vi "WaitOnStopMove.vi"(8 "error in (no error)":errorcluster, 9 "ignore previous (F)":bool, 10 "timeout in ms (-1)":i32, 11 "Game in":refnum<class "Game.lvclass">) -> (0 "error out":errorcluster, 2 "timed out?":bool, 3 "Game out":refnum<class "Game.lvclass">)   [LabVIEW 2019, in "RT_Game.lvlib" / "Game.lvclass"]
uses:
  Game.lvclass
  Game.lvclass/Game.ctl
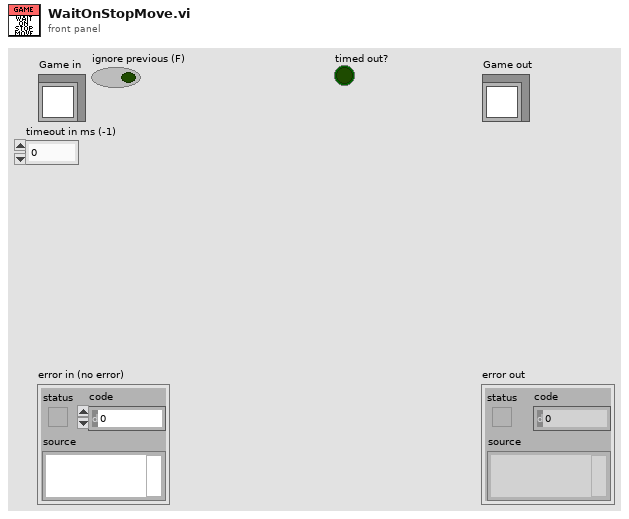
[diagram p1: front panel]
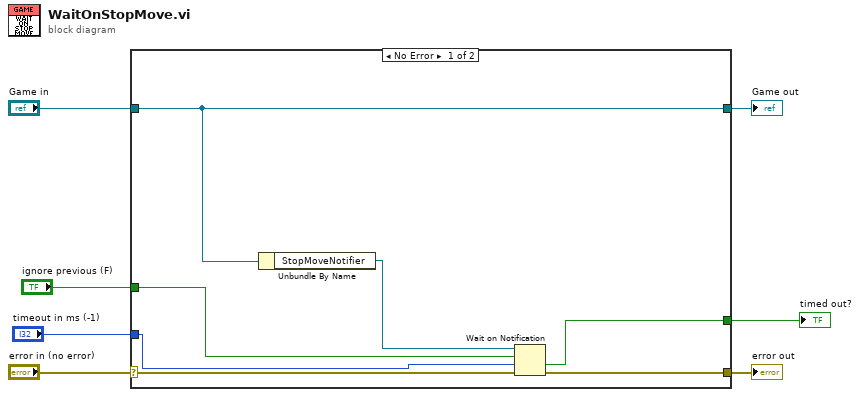
[diagram p0: block diagram]
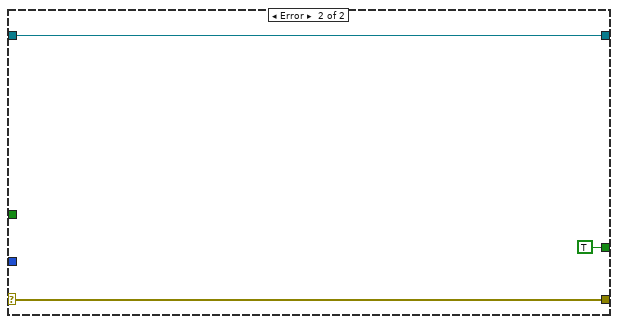
[diagram p2: hidden frame]
diagram:
  n1 = case shown="No Error" "error in (no error)" {
    selector: "error in (no error)" -> [w14 w17]
    tunnel: [w13 w17] -> w6
    tunnel: [w12 w16] -> w4
    tunnel: "Game in" -> [w12 w16]
    tunnel: "timeout in ms (-1)" -> [w10 _]
    tunnel: "ignore previous (F)" -> [w9 _]
    tunnel: [w8 TRUE ("timed out?")] -> w1
    frame No Error {
      n2 = Unbundle By Name(w12) -> ("StopMoveNotifier"=w11:refnum<notifier>)
      n3 = Wait on Notification(notifier=w11, ignore previous (F)=w9, timeout in ms (-1)=w10, error in (no error)=w14) -> (timed out?=w8:bool, error out=w13:errorcluster)  [unwired: 2 out]
    }
    frame Error {
    }
  }
  "error out" <- w6
  "Game out" <- w4
  "timed out?" <- w1
